vi "CAN close.vi"(4 "error in (no error)":errorcluster, 7 "CANopen in":refnum<class "CANopen.lvclass">) -> (0 "error out":errorcluster)   [LabVIEW 2017, in "canopen.lvlib" / "CANopen.lvclass"]
doc: "Closes a previously established connection, freeing every allocated resouce. The closing step is executed independently of the error condition on input. The error out is a merge of the error in and the error returned by the close operation."
uses:
  CANopen.lvclass
  CANopen.lvclass/CANopen.ctl
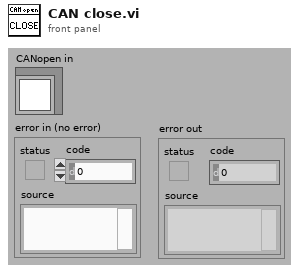
[diagram p1: front panel]
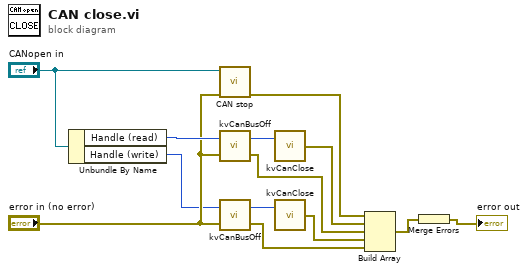
[diagram p0: block diagram]
diagram:
  n1 = Unbundle By Name("CANopen in") -> ("Handle (read)"=w13:i32, "Handle (write)"=w9:i32)
  n2 = call "CAN stop.vi"("error in (no error)"="error in (no error)", "CANopen in"="CANopen in") -> ("error out"=w2:errorcluster)  [unwired: 5 out]
  n3 = call <userlib>:"kvCanBusOff.vi"("error in (no error)"="error in (no error)", "Channel Handle (input only)"=w13) -> ("error out"=w1:errorcluster, "Channel Handle (ouput only)"=w12:i32)
  n4 = call <userlib>:"kvCanBusOff.vi"("error in (no error)"="error in (no error)", "Channel Handle (input only)"=w9) -> ("error out"=w7:errorcluster, "Channel Handle (ouput only)"=w6:i32)
  n5 = call <userlib>:"kvCanClose.vi"("Channel Handle (input only)"=w12) -> ("error out"=w5:errorcluster)  [unwired: 1 in]
  n6 = call <userlib>:"kvCanClose.vi"("Channel Handle (input only)"=w6) -> ("error out"=w8:errorcluster)  [unwired: 1 in]
  n7 = Build Array(w2, w5, w1, w8, w7) -> (w3:errorcluster[])
  n8 = Merge Errors(w3) -> (→"error out":errorcluster)
